vi "user input.vi"(8 "error in":errorcluster, 11 "FPGA Interface":T1) -> (0 "error out":errorcluster, 3 "Inputs from system":T2)   [LabVIEW 2017, in "GPIC Core runtime.lvclass"]
uses:
  GPIC Core runtime.lvclass
  input user data.ctl
  CoreControlsRef.ctl
  <vilib>/Utility/error.llb/Error Cluster From Error Code.vi
  <vilib>/rvi/errors/niLvFpgaAdjustHostInterfaceError.vi
  <vilib>/rvi/interface/nirviReadWriteControl/nirviReadWriteControl.xnode
  NiFpgaLv.dll
  <vilib>/rvi/interface/Simulation/niFpgaSimulationCallBeginRW.vi
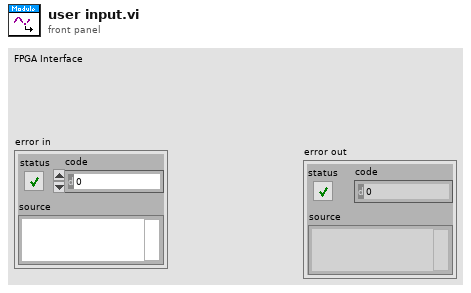
[diagram p1: front panel]
types:
  T1 = typedef "GPIC Core runtime.lvclass/CoreControlsRef.ctl" = refnum<k20>
  T2 = typedef "GPIC Core runtime.lvclass/input user data.ctl" = cluster{"AO_AO0":i16, "AO_AO1":i16, "AO_AO2":i16, "AO_AO3":i16, "AO_AO4":i16, "AO_AO5":i16, "AO_AO6":i16, "AO_AO7":i16, "HalfBridge_DO0":bool, "HalfBridge_DO1":bool, "HalfBridge_DO2":bool, "HalfBridge_DO3":bool, "HalfBridge_DO4":bool, "HalfBridge_DO5":bool, "HalfBridge_DO6":bool, "HalfBridge_DO7":bool, "HalfBridge_DO8":bool, "HalfBridge_DO9":bool, "HalfBridge_DO10":bool, "HalfBridge_DO11":bool, "HalfBridge_DO12":bool, "HalfBridge_DO13":bool, "LVTTL_DIO0":bool, "LVTTL_DIO1":bool, "LVTTL_DIO2":bool, "LVTTL_DIO3":bool, "LVTTL_DIO4":bool, "LVTTL_DIO5":bool, "LVTTL_DIO6":bool, "LVTTL_DIO7":bool, "LVTTL_DIO8":bool, "LVTTL_DIO9":bool, "LVTTL_DIO10":bool, "LVTTL_DIO11":bool, "LVTTL_DIO12":bool, "LVTTL_DIO13":bool, "LVTTL_DIO14":bool, "LVTTL_DIO15":bool, "LVTTL_DIO16":bool, "LVTTL_DIO17":bool, "LVTTL_DIO18":bool, "LVTTL_DIO19":bool, "LVTTL_DIO20":bool, "LVTTL_DIO21":bool, "LVTTL_DIO22":bool, "LVTTL_DIO23":bool, "LVTTL_DIO24":bool, "LVTTL_DIO25":bool, "LVTTL_DIO26":bool, "LVTTL_DIO27":bool, "LVTTL_DIO28":bool, "LVTTL_DIO29":bool, "LVTTL_DIO30":bool, "LVTTL_DIO31":bool, "RelayControl_DO0":bool, "RelayControl_DO1":bool, "RelayContro_DOl2":bool, "RelayControl_DO3":bool, "Scanned_AI0":sgl, "Scanned_AI1":sgl, "Scanned_AI2":sgl, "Scanned_AI3":sgl, "Scanned_AI4":sgl, "Scanned_AI5":sgl, "Scanned_AI6":sgl, "Scanned_AI7":sgl, "Simultaneous_AI0":sgl, "Simultaneous_AI1":sgl, "Simultaneous_AI2":sgl, "Simultaneous_AI3":sgl, "Simultaneous_AI4":sgl, "Simultaneous_AI5":sgl, "Simultaneous_AI6":sgl, "Simultaneous_AI7":sgl, "Simultaneous_AI8":sgl, "Simultaneous_AI9":sgl, "Simultaneous_AI10":sgl, "Simultaneous_AI11":sgl, "Simultaneous_AI12":sgl, "Simultaneous_AI13":sgl, "Simultaneous_AI14":sgl, "Simultaneous_AI15":sgl, "Sinking_DO0":bool, "Sinking_DO1":bool, "Sinking_DO2":bool, "Sinking_DO3":bool, "Sinking_DO4":bool, "Sinking_DO5":bool, "Sinking_DO6":bool, "Sinking_DO7":bool, "Sinking_DO8":bool, "Sinking_DO9":bool, "Sinking_DO10":bool, "Sinking_DO11":bool, "Sinking_DO12":bool, "Sinking_DO13":bool, "Sinking_DO14":bool, "Sinking_DO15":bool, "Sinking_DO16":bool, "Sinking_DO17":bool, "Sinking_DO18":bool, "Sinking_DO19":bool, "Sinking_DO20":bool, "Sinking_DO21":bool, "Sinking_DO22":bool, "Sinking_DO23":bool, "Sourcing_P0_DI0":bool, "Sourcing_P0_DI1":bool, "Sourcing_P0_DI2":bool, "Sourcing_P0_DI3":bool, "Sourcing_P0_DI4":bool, "Sourcing_P0_DI5":bool, "Sourcing_P0_DI6":bool, "Sourcing_P0_DI7":bool, "Sourcing_P0_DI8":bool, "Sourcing_P0_DI9":bool, "Sourcing_P0_DI10":bool, "Sourcing_P0_DI11":bool, "Sourcing_P0_DI12":bool, "Sourcing_P0_DI13":bool, "Sourcing_P1_DI0":bool, "Sourcing_P1_DI1":bool, "Sourcing_P1_DI2":bool, "Sourcing_P1_DI3":bool, "Sourcing_P1_DI4":bool, "Sourcing_P1_DI5":bool, "Sourcing_P1_DI6":bool, "Sourcing_P1_DI7":bool, "Sourcing_P1_DI8":bool, "Sourcing_P1_DI9":bool, "Sourcing_P1_DI10":bool, "Sourcing_P1_DI11":bool, "Sourcing_P1_DI12":bool, "Sourcing_P1_DI13":bool}
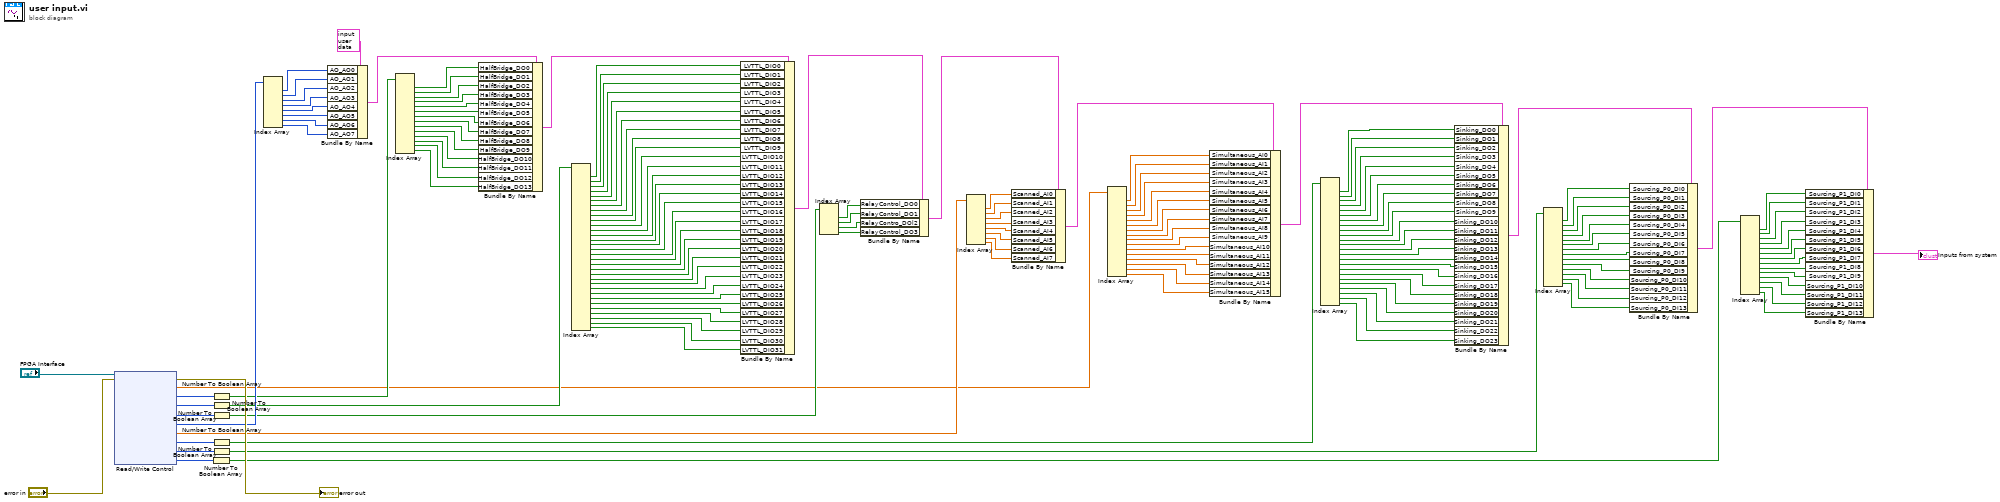
[diagram p0: block diagram]
diagram:
  n1 = xnode "Read/Write Control"("FPGA VI Reference In"="FPGA Interface", "error in"="error in") -> ("error out"=→"error out":errorcluster, "Simultaneous_AI"=w79:sgl[], "HalfBridge"=w150:u16, "LVTTL_DIO"=w131:u32, "RelayControl_DO"=w96:u8, "AO"=w141:i16[], "Scanned_AI"=w89:sgl[], "Sinking_DO"=w61:u32, "Sourcing_P0_DI"=w35:u16, "Sourcing_P1_DI"=w17:u16)  [unwired: 1 out]
  n2 = Number To Boolean Array(number=w17) -> (Boolean array=w16:bool[])
  n3 = Number To Boolean Array(number=w150) -> (Boolean array=w140:bool[])
  n4 = Number To Boolean Array(number=w131) -> (Boolean array=w130:bool[])
  n5 = Number To Boolean Array(number=w96) -> (Boolean array=w95:bool[])
  n6 = Number To Boolean Array(number=w61) -> (Boolean array=w60:bool[])
  n7 = Number To Boolean Array(number=w35) -> (Boolean array=w34:bool[])
  n8 = Index Array(array=w141) -> (element #1=w158:i16, element #2=w157:i16, element #3=w156:i16, element #4=w155:i16, element #5=w154:i16, element #6=w153:i16, element #7=w152:i16, element #8=w151:i16)  [unwired: 8 in]
  n9 = Bundle By Name(cluster=T2 {"AO_AO0"=0, "AO_AO1"=0, "AO_AO2"=0, "AO_AO3"=0, "AO_AO4"=0, "AO_AO5"=0, "AO_AO6"=0, "AO_AO7"=0, "HalfBridge_DO0"=FALSE, "HalfBridge_DO1"=FALSE, "HalfBridge_DO2"=FALSE, "HalfBridge_DO3"=FALSE, "HalfBridge_DO4"=FALSE, "HalfBridge_DO5"=FALSE, "HalfBridge_DO6"=FALSE, "HalfBridge_DO7"=FALSE, "HalfBridge_DO8"=FALSE, "HalfBridge_DO9"=FALSE, "HalfBridge_DO10"=FALSE, "HalfBridge_DO11"=FALSE, "HalfBridge_DO12"=FALSE, "HalfBridge_DO13"=FALSE, "LVTTL_DIO0"=FALSE, "LVTTL_DIO1"=FALSE, "LVTTL_DIO2"=FALSE, "LVTTL_DIO3"=FALSE, "LVTTL_DIO4"=FALSE, "LVTTL_DIO5"=FALSE, "LVTTL_DIO6"=FALSE, "LVTTL_DIO7"=FALSE, "LVTTL_DIO8"=FALSE, "LVTTL_DIO9"=FALSE, "LVTTL_DIO10"=FALSE, "LVTTL_DIO11"=FALSE, "LVTTL_DIO12"=FALSE, "LVTTL_DIO13"=FALSE, "LVTTL_DIO14"=FALSE, "LVTTL_DIO15"=FALSE, "LVTTL_DIO16"=FALSE, "LVTTL_DIO17"=FALSE, "LVTTL_DIO18"=FALSE, "LVTTL_DIO19"=FALSE, "LVTTL_DIO20"=FALSE, "LVTTL_DIO21"=FALSE, "LVTTL_DIO22"=FALSE, "LVTTL_DIO23"=FALSE, "LVTTL_DIO24"=FALSE, "LVTTL_DIO25"=FALSE, "LVTTL_DIO26"=FALSE, "LVTTL_DIO27"=FALSE, "LVTTL_DIO28"=FALSE, "LVTTL_DIO29"=FALSE, "LVTTL_DIO30"=FALSE, "LVTTL_DIO31"=FALSE, "RelayControl_DO0"=FALSE, "RelayControl_DO1"=FALSE, "RelayContro_DOl2"=FALSE, "RelayControl_DO3"=FALSE, "Scanned_AI0"=0.0, "Scanned_AI1"=0.0, "Scanned_AI2"=0.0, "Scanned_AI3"=0.0, "Scanned_AI4"=0.0, "Scanned_AI5"=0.0, "Scanned_AI6"=0.0, "Scanned_AI7"=0.0, "Simultaneous_AI0"=0.0, "Simultaneous_AI1"=0.0, "Simultaneous_AI2"=0.0, "Simultaneous_AI3"=0.0, "Simultaneous_AI4"=0.0, "Simultaneous_AI5"=0.0, "Simultaneous_AI6"=0.0, "Simultaneous_AI7"=0.0, "Simultaneous_AI8"=0.0, "Simultaneous_AI9"=0.0, "Simultaneous_AI10"=0.0, "Simultaneous_AI11"=0.0, "Simultaneous_AI12"=0.0, "Simultaneous_AI13"=0.0, "Simultaneous_AI14"=0.0, "Simultaneous_AI15"=0.0, "Sinking_DO0"=FALSE, "Sinking_DO1"=FALSE, "Sinking_DO2"=FALSE, "Sinking_DO3"=FALSE, "Sinking_DO4"=FALSE, "Sinking_DO5"=FALSE, "Sinking_DO6"=FALSE, "Sinking_DO7"=FALSE, "Sinking_DO8"=FALSE, "Sinking_DO9"=FALSE, "Sinking_DO10"=FALSE, "Sinking_DO11"=FALSE, "Sinking_DO12"=FALSE, "Sinking_DO13"=FALSE, "Sinking_DO14"=FALSE, "Sinking_DO15"=FALSE, "Sinking_DO16"=FALSE, "Sinking_DO17"=FALSE, "Sinking_DO18"=FALSE, "Sinking_DO19"=FALSE, "Sinking_DO20"=FALSE, "Sinking_DO21"=FALSE, "Sinking_DO22"=FALSE, "Sinking_DO23"=FALSE, "Sourcing_P0_DI0"=FALSE, "Sourcing_P0_DI1"=FALSE, "Sourcing_P0_DI2"=FALSE, "Sourcing_P0_DI3"=FALSE, "Sourcing_P0_DI4"=FALSE, "Sourcing_P0_DI5"=FALSE, "Sourcing_P0_DI6"=FALSE, "Sourcing_P0_DI7"=FALSE, "Sourcing_P0_DI8"=FALSE, "Sourcing_P0_DI9"=FALSE, "Sourcing_P0_DI10"=FALSE, "Sourcing_P0_DI11"=FALSE, "Sourcing_P0_DI12"=FALSE, "Sourcing_P0_DI13"=FALSE, "Sourcing_P1_DI0"=FALSE, "Sourcing_P1_DI1"=FALSE, "Sourcing_P1_DI2"=FALSE, "Sourcing_P1_DI3"=FALSE, "Sourcing_P1_DI4"=FALSE, "Sourcing_P1_DI5"=FALSE, "Sourcing_P1_DI6"=FALSE, "Sourcing_P1_DI7"=FALSE, "Sourcing_P1_DI8"=FALSE, "Sourcing_P1_DI9"=FALSE, "Sourcing_P1_DI10"=FALSE, "Sourcing_P1_DI11"=FALSE, "Sourcing_P1_DI12"=FALSE, "Sourcing_P1_DI13"=FALSE} ("Inputs from system"), "AO_AO0"=w158, "AO_AO1"=w157, "AO_AO2"=w156, "AO_AO3"=w155, "AO_AO4"=w154, "AO_AO5"=w153, "AO_AO6"=w152, "AO_AO7"=w151) -> (w139:T2)
  n10 = Index Array(array=w140) -> (element #1=w149:bool, element #2=w148:bool, element #3=w147:bool, element #4=w146:bool, element #5=w145:bool, element #6=w144:bool, element #7=w143:bool, element #8=w142:bool, element #9=w137:bool, element #10=w136:bool, element #11=w135:bool, element #12=w134:bool, element #13=w133:bool, element #14=w132:bool)  [unwired: 14 in]
  n11 = Bundle By Name(cluster=w139, "HalfBridge_DO0"=w149, "HalfBridge_DO1"=w148, "HalfBridge_DO2"=w147, "HalfBridge_DO3"=w146, "HalfBridge_DO4"=w145, "HalfBridge_DO5"=w144, "HalfBridge_DO6"=w143, "HalfBridge_DO7"=w142, "HalfBridge_DO8"=w137, "HalfBridge_DO9"=w136, "HalfBridge_DO10"=w135, "HalfBridge_DO11"=w134, "HalfBridge_DO12"=w133, "HalfBridge_DO13"=w132) -> (w138:T2)
  n12 = Index Array(array=w130) -> (element #1=w129:bool, element #2=w128:bool, element #3=w127:bool, element #4=w126:bool, element #5=w125:bool, element #6=w124:bool, element #7=w123:bool, element #8=w122:bool, element #9=w121:bool, element #10=w120:bool, element #11=w119:bool, element #12=w118:bool, element #13=w117:bool, element #14=w116:bool, element #15=w115:bool, element #16=w114:bool, element #17=w113:bool, element #18=w112:bool, element #19=w111:bool, element #20=w110:bool, element #21=w109:bool, element #22=w108:bool, element #23=w107:bool, element #24=w106:bool, element #25=w105:bool, element #26=w104:bool, element #27=w103:bool, element #28=w102:bool, element #29=w101:bool, element #30=w100:bool, element #31=w99:bool, element #32=w98:bool)  [unwired: 32 in]
  n13 = Bundle By Name(cluster=w138, "LVTTL_DIO0"=w129, "LVTTL_DIO1"=w128, "LVTTL_DIO2"=w127, "LVTTL_DIO3"=w126, "LVTTL_DIO4"=w125, "LVTTL_DIO5"=w124, "LVTTL_DIO6"=w123, "LVTTL_DIO7"=w122, "LVTTL_DIO8"=w121, "LVTTL_DIO9"=w120, "LVTTL_DIO10"=w119, "LVTTL_DIO11"=w118, "LVTTL_DIO12"=w117, "LVTTL_DIO13"=w116, "LVTTL_DIO14"=w115, "LVTTL_DIO15"=w114, "LVTTL_DIO16"=w113, "LVTTL_DIO17"=w112, "LVTTL_DIO18"=w111, "LVTTL_DIO19"=w110, "LVTTL_DIO20"=w109, "LVTTL_DIO21"=w108, "LVTTL_DIO22"=w107, "LVTTL_DIO23"=w106, "LVTTL_DIO24"=w105, "LVTTL_DIO25"=w104, "LVTTL_DIO26"=w103, "LVTTL_DIO27"=w102, "LVTTL_DIO28"=w101, "LVTTL_DIO29"=w100, "LVTTL_DIO30"=w99, "LVTTL_DIO31"=w98) -> (w97:T2)
  n14 = Index Array(array=w95) -> (element #1=w94:bool, element #2=w93:bool, element #3=w92:bool, element #4=w91:bool)  [unwired: 4 in]
  n15 = Bundle By Name(cluster=w97, "RelayControl_DO0"=w94, "RelayControl_DO1"=w93, "RelayContro_DOl2"=w92, "RelayControl_DO3"=w91) -> (w90:T2)
  n16 = Index Array(array=w89) -> (element #1=w88:sgl, element #2=w87:sgl, element #3=w86:sgl, element #4=w85:sgl, element #5=w84:sgl, element #6=w83:sgl, element #7=w82:sgl, element #8=w81:sgl)  [unwired: 8 in]
  n17 = Bundle By Name(cluster=w90, "Scanned_AI0"=w88, "Scanned_AI1"=w87, "Scanned_AI2"=w86, "Scanned_AI3"=w85, "Scanned_AI4"=w84, "Scanned_AI5"=w83, "Scanned_AI6"=w82, "Scanned_AI7"=w81) -> (w80:T2)
  n18 = Index Array(array=w79) -> (element #1=w78:sgl, element #2=w77:sgl, element #3=w76:sgl, element #4=w75:sgl, element #5=w74:sgl, element #6=w73:sgl, element #7=w72:sgl, element #8=w71:sgl, element #9=w70:sgl, element #10=w69:sgl, element #11=w68:sgl, element #12=w67:sgl, element #13=w66:sgl, element #14=w65:sgl, element #15=w64:sgl, element #16=w63:sgl)  [unwired: 16 in]
  n19 = Bundle By Name(cluster=w80, "Simultaneous_AI0"=w78, "Simultaneous_AI1"=w77, "Simultaneous_AI2"=w76, "Simultaneous_AI3"=w75, "Simultaneous_AI4"=w74, "Simultaneous_AI5"=w73, "Simultaneous_AI6"=w72, "Simultaneous_AI7"=w71, "Simultaneous_AI8"=w70, "Simultaneous_AI9"=w69, "Simultaneous_AI10"=w68, "Simultaneous_AI11"=w67, "Simultaneous_AI12"=w66, "Simultaneous_AI13"=w65, "Simultaneous_AI14"=w64, "Simultaneous_AI15"=w63) -> (w62:T2)
  n20 = Index Array(array=w60) -> (element #1=w59:bool, element #2=w58:bool, element #3=w57:bool, element #4=w56:bool, element #5=w55:bool, element #6=w54:bool, element #7=w53:bool, element #8=w52:bool, element #9=w51:bool, element #10=w50:bool, element #11=w49:bool, element #12=w48:bool, element #13=w47:bool, element #14=w46:bool, element #15=w45:bool, element #16=w44:bool, element #17=w43:bool, element #18=w42:bool, element #19=w41:bool, element #20=w40:bool, element #21=w39:bool, element #22=w38:bool, element #23=w37:bool, element #24=w36:bool)  [unwired: 24 in]
  n21 = Bundle By Name(cluster=w62, "Sinking_DO0"=w59, "Sinking_DO1"=w58, "Sinking_DO2"=w57, "Sinking_DO3"=w56, "Sinking_DO4"=w55, "Sinking_DO5"=w54, "Sinking_DO6"=w53, "Sinking_DO7"=w52, "Sinking_DO8"=w51, "Sinking_DO9"=w50, "Sinking_DO10"=w49, "Sinking_DO11"=w48, "Sinking_DO12"=w47, "Sinking_DO13"=w46, "Sinking_DO14"=w45, "Sinking_DO15"=w44, "Sinking_DO16"=w43, "Sinking_DO17"=w42, "Sinking_DO18"=w41, "Sinking_DO19"=w40, "Sinking_DO20"=w39, "Sinking_DO21"=w38, "Sinking_DO22"=w37, "Sinking_DO23"=w36) -> (w33:T2)
  n22 = Index Array(array=w34) -> (element #1=w32:bool, element #2=w31:bool, element #3=w30:bool, element #4=w29:bool, element #5=w28:bool, element #6=w27:bool, element #7=w26:bool, element #8=w25:bool, element #9=w24:bool, element #10=w23:bool, element #11=w22:bool, element #12=w21:bool, element #13=w20:bool, element #14=w19:bool)  [unwired: 14 in]
  n23 = Bundle By Name(cluster=w33, "Sourcing_P0_DI0"=w32, "Sourcing_P0_DI1"=w31, "Sourcing_P0_DI2"=w30, "Sourcing_P0_DI3"=w29, "Sourcing_P0_DI4"=w28, "Sourcing_P0_DI5"=w27, "Sourcing_P0_DI6"=w26, "Sourcing_P0_DI7"=w25, "Sourcing_P0_DI8"=w24, "Sourcing_P0_DI9"=w23, "Sourcing_P0_DI10"=w22, "Sourcing_P0_DI11"=w21, "Sourcing_P0_DI12"=w20, "Sourcing_P0_DI13"=w19) -> (w18:T2)
  n24 = Index Array(array=w16) -> (element #1=w15:bool, element #2=w14:bool, element #3=w13:bool, element #4=w12:bool, element #5=w11:bool, element #6=w10:bool, element #7=w9:bool, element #8=w8:bool, element #9=w7:bool, element #10=w6:bool, element #11=w5:bool, element #12=w4:bool, element #13=w3:bool, element #14=w2:bool)  [unwired: 14 in]
  n25 = Bundle By Name(cluster=w18, "Sourcing_P1_DI0"=w15, "Sourcing_P1_DI1"=w14, "Sourcing_P1_DI2"=w13, "Sourcing_P1_DI3"=w12, "Sourcing_P1_DI4"=w11, "Sourcing_P1_DI5"=w10, "Sourcing_P1_DI6"=w9, "Sourcing_P1_DI7"=w8, "Sourcing_P1_DI8"=w7, "Sourcing_P1_DI9"=w6, "Sourcing_P1_DI10"=w5, "Sourcing_P1_DI11"=w4, "Sourcing_P1_DI12"=w3, "Sourcing_P1_DI13"=w2) -> (→"Inputs from system":T2)
